vi "PH_Get6PInformation.get and prepare Info.vi"(5 "error in":errorcluster) -> (14 "ColHdrs[]":string[](array[string])=["Sixpack Instance", "Axis"], 15 "RowHdrs[]":string[](array[string]), 16 "ItemNames":string[][](array[string]), 17 "Row Cell BG":u32[](array[numeric]), 18 "Rows with GUI conflict":i32[](array[numeric]), 19 "error out":errorcluster)   [LabVIEW 2014, in "PH_Get6PInformation.lvlib"]
doc: "This VI is reading out information from the database and prepares it for the visualisation on the GUI."
uses:
  PH_Get6PInformation.lvlib
  PH_Basics/PH_Stepmotor_BaseClass/PH_Stepmotor_BaseClass.Motor Type.ctl
  PH_Basics/PH_Stepmotor_BaseClass/PH_Stepmotor_BaseClass.Axis Address.ctl
  PH_Basics/PH_Common/PH_Common.lvlib
  PH_Basics/PH_Stepmotor_BaseClass/PH_Stepmotor_BaseClass.lvlib
  PH_Devices/PH_Sixpack/PH_Sixpack.lvlib
  PH_Devices/PH_Beckhoff/PH_Beckhoff.lvlib
  PH_Basics/PH_AxisGUI_BaseClass/PH_AxisGUI_BaseClass.lvlib
panel:
  in  "Type":T1
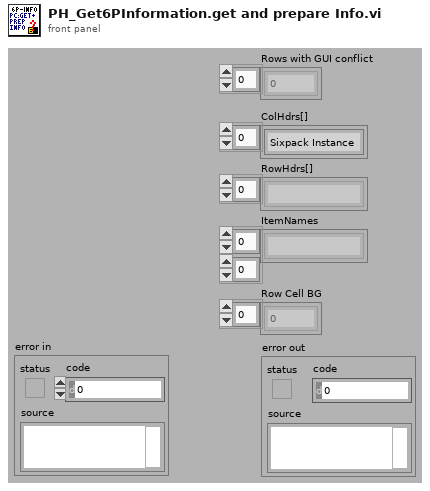
[diagram p1: front panel]
types:
  T1 = typedef "PH_Stepmotor_BaseClass.lvlib/PH_Stepmotor_BaseClass.Motor Type.ctl" = enum16{"Unspecific", "OWIS 49.120.2633", "OWIS 49.060.1033", "OWIS 43.040.2558", "Diamond Motion 2200 series", "OWIS 49.120.266B.MV6", "Calorimeter", "Linear Stage 1", "MICOS VT-80", "MICOS VT-80 S", "Standa Rotstage nt0.95A", "PUF RA 320.200", "PUF RA 800.200", "PUF RA 800.400", "PUF RA 400.50", "1324.nn.800.50", "1324.n9c.800.50", "1324.nn.320.200", "1324.nn.400.200", "1324.nn.800.200", "1324.nn.400.50", "1324.8c9c.800.50", "1324.8c9c.400.200"}
  T2 = typedef "PH_Stepmotor_BaseClass.lvlib/PH_Stepmotor_BaseClass.Axis Address.ctl" = cluster{"Instance":string, "Motor Nr":i32}
  T3 = cluster{"Address":T2, "GUI Class":string, "GUI Instance":string}[]
  T4 = cluster{"Address":T2, "GUI Class":string, "GUI Instance":string}
  T5 = typedef "PH_Stepmotor_BaseClass.lvlib/PH_Stepmotor_BaseClass.Axis Settings.ctl" = cluster{"Sign change":bool, "Width":dbl, "Calibration":dbl, "Unit":string, "Motor Type":T1, "Unit Width":string, "Unit CF":string}
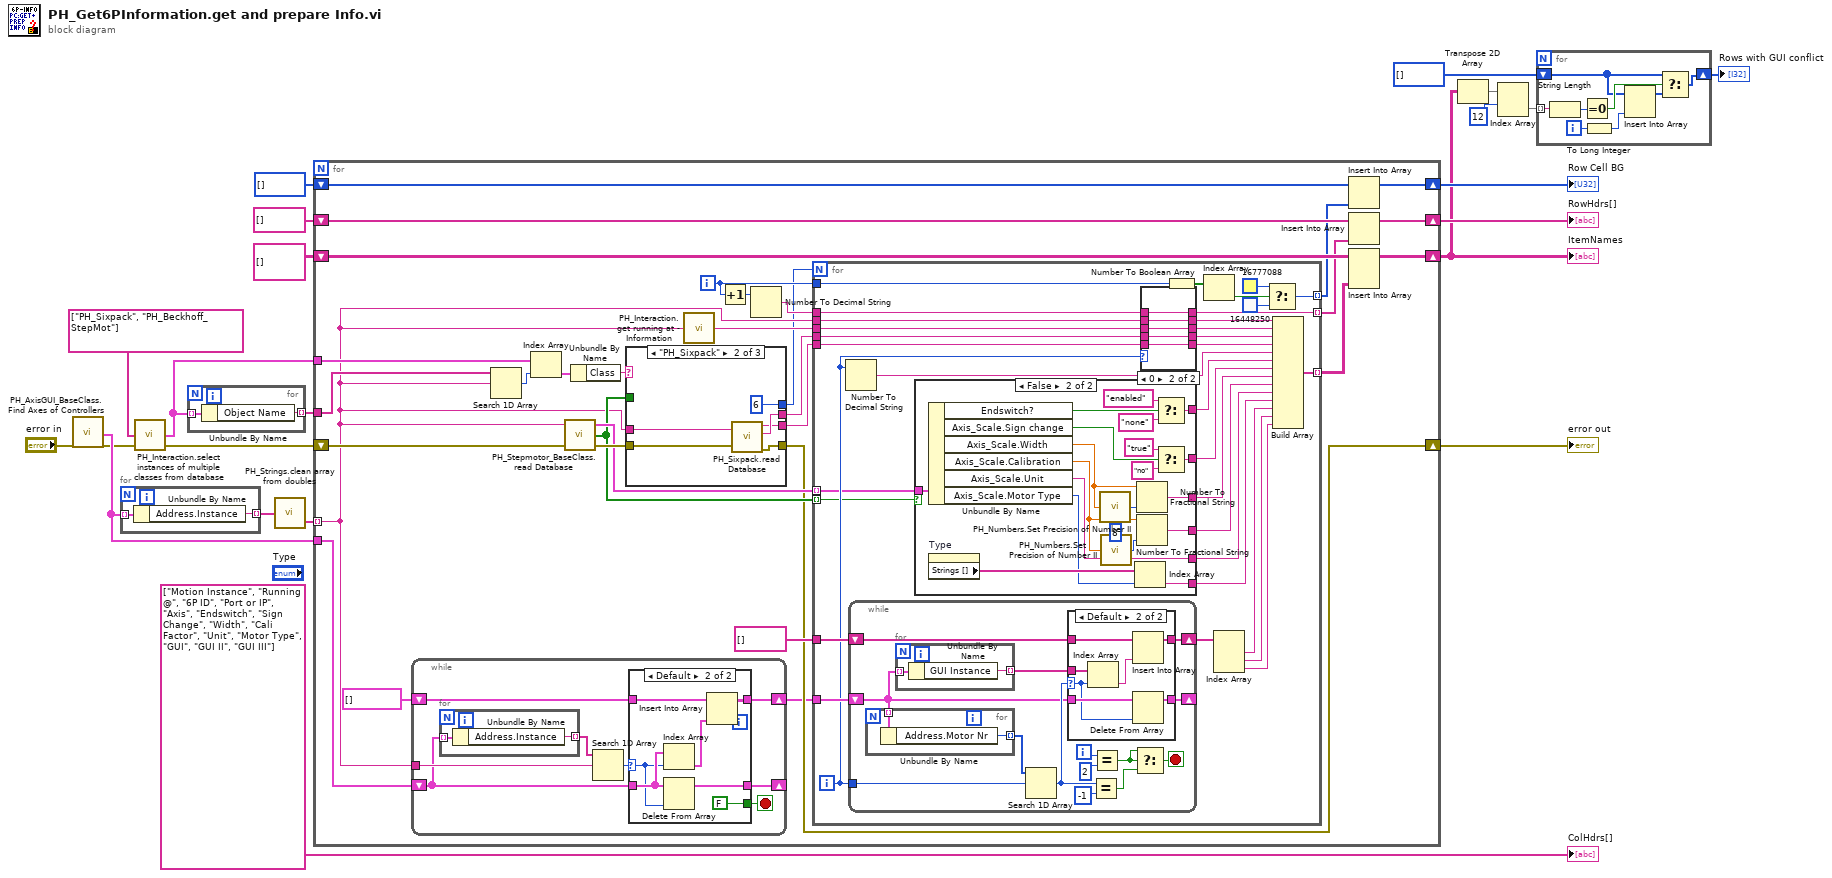
[diagram p0: block diagram]
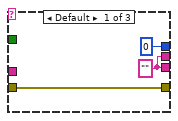
[diagram p2: hidden frame]
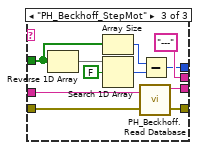
[diagram p3: hidden frame]
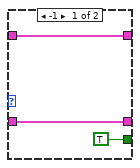
[diagram p4: hidden frame]
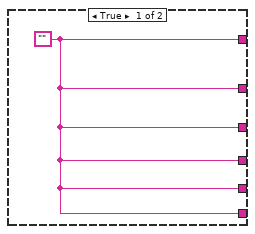
[diagram p5: hidden frame]
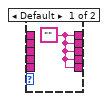
[diagram p7: hidden frame]
diagram:
  n1 = call "PH_AxisGUI_BaseClass.Find Axes of Controllers.vi"("error in"="error in") -> ("Result"=w13:T3, "error out"=w10:errorcluster)  [unwired: 17 in]
  n2 = for {
    tunnel: w13 -> [w24] mode=indexing
    tunnel: [w23] -> w12 mode=indexing
    n3 = Unbundle By Name(w24) -> ("Address.Instance"=w23:string)
  }
  n4 = call "PH_Interaction.select instances of multiple classes from database.vi"("error in (no error)"=w10, "Classes Input"=string[] ["PH_Sixpack", "PH_Beckhoff_StepMot"]) -> ("error out"=w9:errorcluster, "Query Result"=w14:cluster{"Object Name":string, "Class":string}[])  [unwired: 2 in]
  n5 = for {
    tunnel: w14 -> [w26] mode=indexing
    tunnel: [w25] -> w15 mode=indexing
    n6 = Unbundle By Name(w26) -> ("Object Name"=w25:string)
  }
  n7 = call "PH_Strings.clean array from doubles.vi"("Array Input"=w12) -> ("Cleaned Array Output"=w17:string[])  [unwired: 1 out]
  n8 = for {
    tunnel: w17 -> [w30] mode=indexing
    shift-right: [w57] -> w7
    shift-left: string[][] [] -> [w56]
    shift-right: [w52] -> w21
    shift-left: string[] [] -> [w53]
    shift-right: [w50] -> w22
    shift-left: u32[] [] -> [w49]
    shift-right: [w29] -> w8
    shift-left: w9 -> [w35]
    tunnel: w13 -> [w46]
    tunnel: w15 -> [w36]
    tunnel: w14 -> [w38]
    i -> [w43]
    n9 = while {
      tunnel: w30 -> [w83]
      shift-right: [w82] -> _
      shift-left: w46 -> [w79]
      shift-right: [w84] -> w28
      shift-left: T3 [] ("Result") -> [w85]
      stop <- w80 stop-if-true
      n10 = for {
        tunnel: w79 -> [w87] mode=indexing
        tunnel: [w86] -> w78 mode=indexing
        n11 = Unbundle By Name(w87) -> ("Address.Instance"=w86:string)
      }
      n12 = Search 1D Array(1D array=w78, element=w83) -> (index of element=w81:i32)  [unwired: 1 in]
      n13 = case shown="Default" w81 {
        selector: w81 -> [_ w95]
        tunnel: w85 -> [w90 w93]
        tunnel: [w90 w92] -> w84
        tunnel: [w89 w97] -> w82
        tunnel: w79 -> [w89 w96]
        tunnel: [TRUE FALSE] -> w80
        frame -1 {
        }
        frame Default {
          n14 = Index Array(array=w96, index=w95) -> (element=w91:T4)
          n15 = Delete From Array(array=w96, index=w95) -> (array with subset deleted=w97:T3)  [unwired: 1 in, 1 out]
          n16 = Insert Into Array(array=w93, new element=w91) -> (w92:T3)  [unwired: 1 in]
        }
      }
    }
    n17 = Search 1D Array(1D array=w36, element=w30) -> (index of element=w40:i32)  [unwired: 1 in]
    n18 = Index Array(array=w38, index=w40) -> (element=w39:cluster{"Object Name":string, "Class":string})
    n19 = call "PH_Stepmotor_BaseClass.read Database.vi"("error in (no error)"=w35, "DB Entry to read"=w30) -> ("error out"=w34:errorcluster, "Entry empty?"=w32:bool[], "Axes Data"=w33:cluster{"Axis_Scale":T5, "Endswitch?":bool}[])  [unwired: 1 in]
    n20 = Unbundle By Name(w39) -> ("Class"=w37:string)
    n21 = case shown="\"PH_Sixpack\"" w37 {
      tunnel: [w59 w65 "---"] -> w48
      tunnel: [w59 w64 w76] -> w41
      tunnel: [0 6 w67] -> w27
      tunnel: [w58 w63 w74] -> w29
      tunnel: w34 -> [w58 w62 w75]
      tunnel: w30 -> [_ w61 w73]
      tunnel: w32 -> [_ _ w68]
      frame Default {
        w59 = ""
      }
      frame "PH_Sixpack" {
        n22 = call "PH_Sixpack.read Database.vi"("DB Entry to read"=w61, "error in (no error)"=w62) -> ("COM Port"=w64:string, "SixPack ID"=w65:string, "error out"=w63:errorcluster)  [unwired: 1 out]
      }
      frame "PH_Beckhoff_StepMot" {
        n23 = Reverse 1D Array(array=w68) -> (reversed array=w69:bool[])
        n24 = Array Size(array=w68) -> (size(s)=w71:i32)
        n25 = Search 1D Array(1D array=w69, element=FALSE) -> (index of element=w72:i32)  [unwired: 1 in]
        n26 = call "PH_Beckhoff.Read Database.vi"("error in (no error)"=w75, "DB Entry to read"=w73) -> ("error out"=w74:errorcluster, "IP"=w76:string)
        n27 = Subtract(x=w71, y=w72) -> (x-y=w67:i32)
      }
    }
    n28 = call "PH_Interaction.get running at - Information.vi"("Instance"=w30) -> ("Running @ - Information"=w47:string)
    n29 = Increment(x=w43) -> (x+1=w42:i32)
    n30 = Number To Decimal String(number=w42) -> (decimal integer string=w55:string)  [unwired: 1 in]
    n31 = for {
      N: w27 -> [_]
      tunnel: w30 -> [w130]
      tunnel: [w128] -> w45 mode=indexing
      tunnel: w55 -> [w127]
      tunnel: [w126] -> w54 mode=indexing
      tunnel: w43 -> [w101]
      tunnel: [w123] -> w51 mode=indexing
      tunnel: w48 -> [w122]
      tunnel: w41 -> [w120]
      tunnel: w47 -> [w111]
      tunnel: string[] [] -> [w109]
      tunnel: w28 -> [w108]
      tunnel: w33 -> [w100] mode=indexing
      tunnel: w32 -> [w98] mode=indexing
      i -> [w104]
      n32 = Number To Decimal String(number=w104) -> (decimal integer string=w102:string)  [unwired: 1 in]
      n33 = while {
        shift-right: [w156] -> _
        shift-left: w108 -> [w154]
        tunnel: w104 -> [w152]
        shift-right: [w164] -> w107
        shift-left: w109 -> [w163]
        i -> [w161]
        stop <- w157 stop-if-true
        n34 = for {
          tunnel: w154 -> [w167] mode=indexing
          tunnel: [w166] -> w153 mode=indexing
          n35 = Unbundle By Name(w167) -> ("Address.Motor Nr"=w166:i32)
        }
        n36 = for {
          tunnel: w154 -> [w169] mode=indexing
          tunnel: [w168] -> w155 mode=indexing
          n37 = Unbundle By Name(w169) -> ("GUI Instance"=w168:string)
        }
        n38 = Search 1D Array(1D array=w153, element=w152) -> (index of element=w162:i32)  [unwired: 1 in]
        n39 = case shown="Default" w162 {
          selector: w162 -> [_ w172]
          tunnel: w155 -> [_ w178]
          tunnel: [w171 w176] -> w164
          tunnel: w163 -> [w171 w175]
          tunnel: [w170 w174] -> w156
          tunnel: w154 -> [w170 w173]
          frame -1 {
          }
          frame Default {
            n40 = Index Array(array=w178, index=w172) -> (element=w177:string)
            n41 = Insert Into Array(array=w175, new element=w177) -> (w176:string[])  [unwired: 1 in]
            n42 = Delete From Array(array=w173, index=w172) -> (array with subset deleted=w174:T3)  [unwired: 1 in, 1 out]
          }
        }
        n43 = Equal?(x=w162, y=-1) -> (x = y?=w158:bool)
        n44 = Equal?(x=w161, y=2 ("x")) -> (x = y?=w159:bool)
        n45 = Select(t=w159, s=w159, f=w158) -> (s? t:f=w157:bool)
      }
      n46 = case shown="False" w98 {
        tunnel: [w131 w149] -> w118
        tunnel: [w131 w148] -> w117
        tunnel: [w131 w147] -> w116
        tunnel: [w131 w146] -> w115
        tunnel: [w131 w145] -> w114
        tunnel: w100 -> [_ w144]
        tunnel: [w131 w133] -> w99
        frame True {
          w131 = ""
        }
        frame False {
          n47 = Unbundle By Name(w144) -> ("Endswitch?"=w143:bool, "Axis_Scale.Sign change"=w136:bool, "Axis_Scale.Width"=w135:dbl, "Axis_Scale.Calibration"=w134:dbl, "Axis_Scale.Unit"=w133:string, "Axis_Scale.Motor Type"=w132:T1)
          n48 = property on="Type" class="Enum (strict)"() -> ("Strings []"=w140:string[])  [unwired: 2 in, 2 out]
          n49 = call "PH_Numbers.Set Precision of Number II.vi"("Number"=w135) -> ("Precision"=w139:i32)  [unwired: 1 in]
          n50 = call "PH_Numbers.Set Precision of Number II.vi"("Number"=w134, "Precision (6)"=u8 8) -> ("Precision"=w138:i32)
          n51 = Index Array(array=w140, index=w132) -> (element=w145:string)
          n52 = Number To Fractional String(number=w135, precision (6)=w139) -> (F-format string=w147:string)  [unwired: 2 in]
          n53 = Number To Fractional String(number=w134, precision (6)=w138) -> (F-format string=w146:string)  [unwired: 2 in]
          n54 = Select(t="enabled" ("element"), s=w143, f="none" ("element")) -> (s? t:f=w149:string)
          n55 = Select(t="true" ("element"), s=w136, f="no" ("element")) -> (s? t:f=w148:string)
        }
      }
      n56 = case shown="0" w104 {
        tunnel: [w179 w184] -> w129
        tunnel: w130 -> [_ w184]
        tunnel: w127 -> [_ w183]
        tunnel: [w179 w183] -> w126
        tunnel: w122 -> [_ w182]
        tunnel: [w179 w182] -> w121
        tunnel: w120 -> [_ w181]
        tunnel: [w179 w181] -> w119
        tunnel: [w179 w180] -> w110
        tunnel: w111 -> [_ w180]
        frame Default {
          w179 = ""
        }
        frame 0 {
        }
      }
      n57 = Number To Boolean Array(number=w101) -> (Boolean array=w124:bool[])
      n58 = Index Array(array=w124) -> (element=w125:bool)  [unwired: 1 in]
      n59 = Index Array(array=w107) -> (element #1=w106:string, element #2=w103:string, element #3=w105:string)  [unwired: 3 in]
      n60 = Select(t=u32 16777088 ("Color Box"), s=w125, f=u32 16448250 ("Color Box")) -> (s? t:f=w123:u32)
      n61 = Build Array(w129, w110, w121, w119, w102, w118, w117, w116, w115, w99, w114, w106, w103, w105) -> (w128:string[])
    }
    n62 = Insert Into Array(array=w49, new element=w51) -> (w50:u32[])  [unwired: 1 in]
    n63 = Insert Into Array(array=w53, new element=w54) -> (w52:string[])  [unwired: 1 in]
    n64 = Insert Into Array(array=w56, new element=w45) -> (w57:string[][])  [unwired: 2 in]
  }
  "error out" <- w8
  "Row Cell BG" <- w22
  "RowHdrs[]" <- w21
  "ItemNames" <- w7
  n65 = Transpose 2D Array(2D array=w7) -> (transposed array=w6:string[][])
  n66 = Index Array(array=w6, index (row)=12) -> (element=w4:string[])  [unwired: 1 in]
  n67 = for {
    tunnel: w4 -> [w192] mode=indexing
    shift-right: [w189] -> w3
    shift-left: i32[] [] -> [w188]
    i -> [w187]
    n68 = String Length(string=w192) -> (length=w191:i32)
    n69 = Equal To 0?(x=w191) -> (x = 0?=w190:bool)
    n70 = To Long Integer(number=w187) -> (32bit integer=w185:i32)
    n71 = Insert Into Array(array=w188, new element=w185) -> (w186:i32[])  [unwired: 1 in]
    n72 = Select(t=w188, s=w190, f=w186) -> (s? t:f=w189:i32[])
  }
  "Rows with GUI conflict" <- w3
  "ColHdrs[]" <- string[] ["Motion Instance", "Running @", "6P ID", "Port or IP", "Axis", "Endswitch", "Sign Change", "Width", "Cali Factor", "Unit", "Motor Type", "GUI", "GUI II", "GUI III"] ("new element/subarray")
